vi "Verify Instrument Options - Versions.vi"(0 "Instrument Info":T1, 5 "Instrument Attributes":T2, 11 "error in (no error)":errorcluster) -> (4 "Options & Versions Validation":string, 6 "Mismatch? (True = Mismatch)":bool, 15 "error out":errorcluster)   [LabVIEW 2018]
uses:
  Controls/Instrument Attributes Cluster.ctl
  Controls/Class Instrument Info.ctl
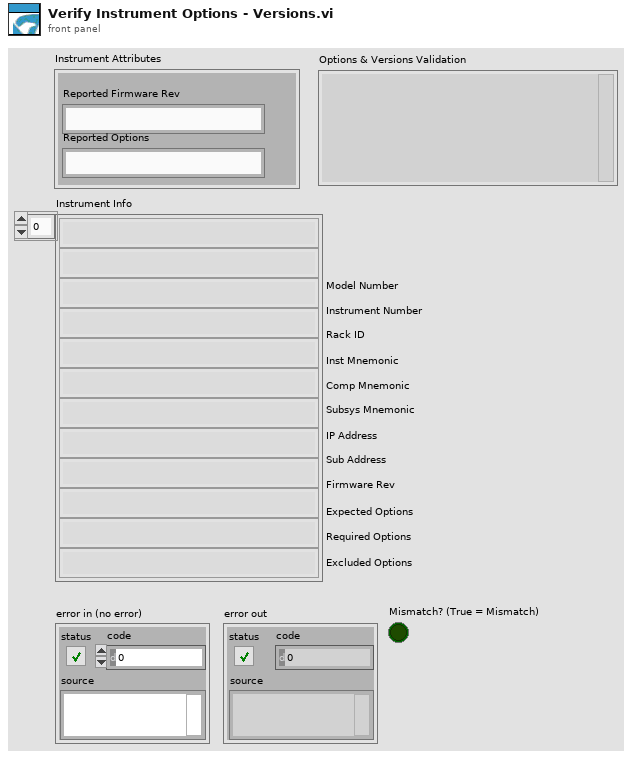
[diagram p1: front panel]
types:
  T1 = typedef "Class Instrument Info.ctl" = string[]
  T2 = typedef "Instrument Attributes Cluster.ctl" = cluster{"Reported Firmware Rev":string, "Reported Options":string}
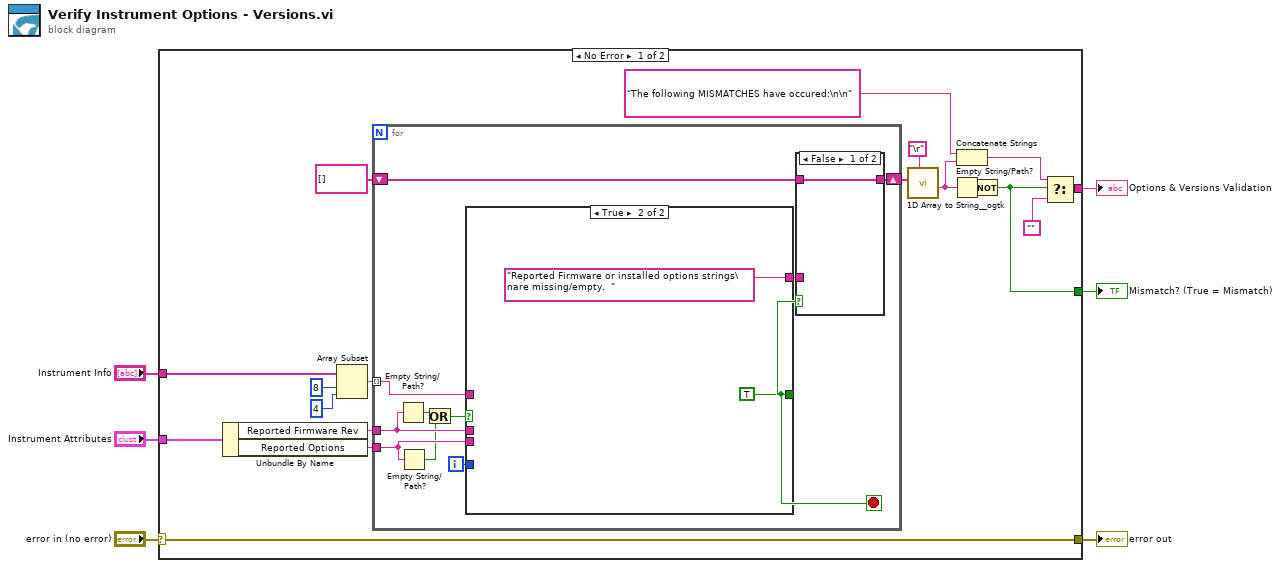
[diagram p0: block diagram]
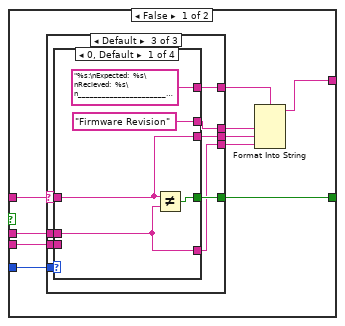
[diagram p2: hidden frame]
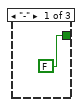
[diagram p3: hidden frame]
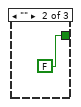
[diagram p4: hidden frame]
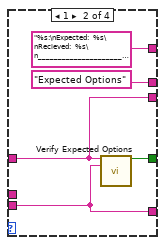
[diagram p5: hidden frame]
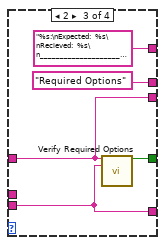
[diagram p6: hidden frame]
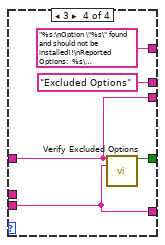
[diagram p7: hidden frame]
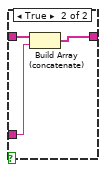
[diagram p8: hidden frame]
diagram:
  n1 = case shown="No Error" "error in (no error)" {
    selector: "error in (no error)" -> [w13 w83]
    tunnel: [w13 w83] -> w5
    tunnel: "Instrument Attributes" -> [w24 _]
    tunnel: "Instrument Info" -> [w23 _]
    tunnel: [w15 _] -> w2
    tunnel: [w10 _] -> w1
    frame No Error {
      n2 = Unbundle By Name(w24) -> ("Reported Firmware Rev"=w8:string, "Reported Options"=w7:string)
      n3 = Array Subset(array=w23, index=8, length=4) -> (w21:T1)
      n4 = for {
        tunnel: w21 -> [w31] mode=indexing
        shift-right: [w34] -> w19
        shift-left: string[] [] -> [w33]
        tunnel: w8 -> [w30]
        tunnel: w7 -> [w29]
        i -> [w32]
        stop <- w25 stop-if-true
        n5 = Empty String/Path?(string/path=w30) -> (empty?=w28:bool)
        n6 = Empty String/Path?(string/path=w29) -> (empty?=w27:bool)
        n7 = Or(x=w28, y=w27) -> (x .or. y?=w26:bool)
        n8 = case shown="True" w26 {
          tunnel: [w45 "Reported Firmware or installed options strings\nare missing/empty.  "] -> w35
          tunnel: w32 -> [w44 _]
          tunnel: w29 -> [w43 _]
          tunnel: [w42 TRUE ("Mismatch? (True = Mismatch)")] -> w25
          tunnel: w31 -> [w38 _]
          tunnel: w30 -> [w36 _]
          frame False {
            n9 = case shown="Default" w38 {
              selector: w38 -> [_ _ w49]
              tunnel: w44 -> [_ _ w56]
              tunnel: w36 -> [_ _ w55]
              tunnel: w43 -> [_ _ w54]
              tunnel: [FALSE FALSE w53] -> w42
              tunnel: [_ _ w52] -> w41
              tunnel: [_ _ w51] -> w40
              tunnel: [_ _ w50] -> w39
              tunnel: [_ _ w48] -> w37
              frame "-" {
              }
              frame "" {
              }
              frame Default {
                n10 = case shown="0, Default" w56 {
                  tunnel: w49 -> [w58 w64 w69 w74]
                  tunnel: w55 -> [w60 _ _ _]
                  tunnel: w54 -> [_ w63 w68 w76]
                  tunnel: [w61 w62 w67 w72] -> w53
                  tunnel: [w60 w63 w68 w76] -> w52
                  tunnel: [w58 w64 w69 w74] -> w51
                  tunnel: ["Firmware Revision" "Expected Options" "Required Options" "Excluded Options"] -> w50
                  tunnel: ["%s:\nExpected:  %s\nRecieved:  %s\n________________________" "%s:\nExpected:  %s\nRecieved:  %s\n________________________" "%s:\nExpected:  %s\nRecieved:  %s\n________________________" "%s:\nOption \"%s\" found and should not be installed!!\nReported Options:  %s\n________________________"] -> w48
                  frame 0, Default {
                    n11 = Not Equal?(x=w58, y=w60) -> (x != y?=w61:bool)
                  }
                  frame 1 {
                    n12 = call "Verify Expected Options.vi"("Expected Options"=w64, "Reported Options"=w63) -> ("Mismatch? (True = Mismatch)"=w62:bool)  [unwired: 12 in, 1 out]
                  }
                  frame 2 {
                    n13 = call "Verify Required Options.vi"("Required Options"=w69, "Reported Options"=w68) -> ("Mismatch? (True = Mismatch)"=w67:bool)  [unwired: 12 in, 1 out]
                  }
                  frame 3 {
                    n14 = call "Verify Excluded Options.vi"("Excluded Options"=w74, "Reported Options"=w76) -> ("Mismatch? (True = Mismatch)"=w72:bool)  [unwired: 12 in, 1 out]
                  }
                }
              }
            }
            n15 = Format Into String(format string=w37, w39, w40, w41) -> (resulting string=w45:string)  [unwired: 2 in, 1 out]
          }
          frame True {
          }
        }
        n16 = case shown="False" w25 {
          tunnel: w35 -> [_ w81]
          tunnel: [w79 w80] -> w34
          tunnel: w33 -> [w79 w82]
          frame False {
          }
          frame True {
            n17 = Build Array (concatenate)(w82, w81) -> (w80:string[])
          }
        }
      }
      n18 = call <userlib>:"1D Array to String__ogtk.vi"("delimiter (Tab)"="\r", "Array of Strings"=w19) -> ("delimited string"=w16:string)  [unwired: 9 in]
      n19 = Empty String/Path?(string/path=w16) -> (empty?=w14:bool)
      n20 = Concatenate Strings("The following MISMATCHES have occured:\n\n", w16) -> (w11:string)
      n21 = Not(x=w14) -> (.not. x?=w10:bool)
      n22 = Select(t=w11, s=w10, f="") -> (s? t:f=w15:string)
    }
    frame Error {
    }
  }
  "error out" <- w5
  "Options & Versions Validation" <- w2
  "Mismatch? (True = Mismatch)" <- w1
